vi "UpdateLoadTroque.vi"(8 "error in (no error)":errorcluster, 10 "TorqueValue(%)":dbl, 11 "MFActor in":refnum<class "MFActor.lvclass">) -> (0 "error out":errorcluster, 3 "MFActor out":refnum<class "MFActor.lvclass">)   [LabVIEW 2024, in "MFActor.lvlib" / "MFActor.lvclass"]
uses:
  MFActor.lvclass
  MFActor.lvclass/MFActor.ctl
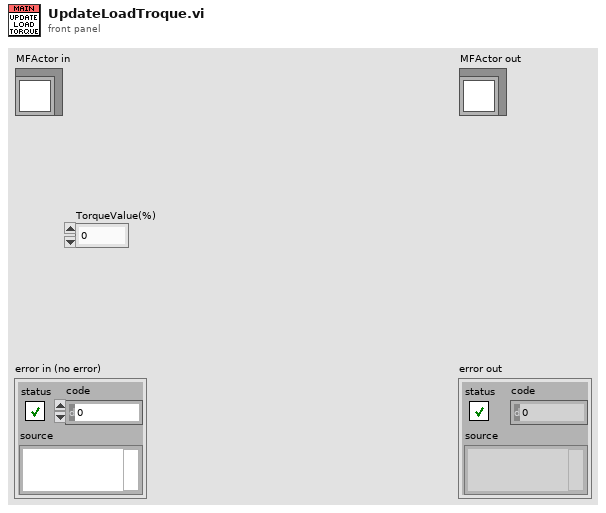
[diagram p1: front panel]
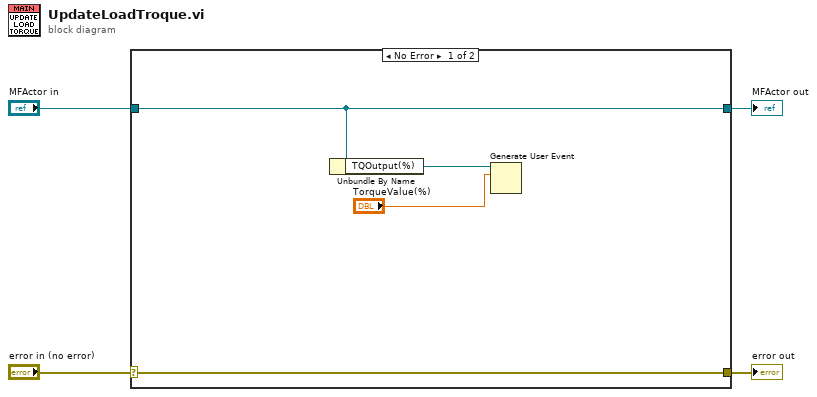
[diagram p0: block diagram]
diagram:
  n1 = case shown="No Error" "error in (no error)" {
    selector: "error in (no error)" -> [w8 w10]
    tunnel: [w8 w10] -> w3
    tunnel: [w7 w9] -> w1
    tunnel: "MFActor in" -> [w7 w9]
    frame No Error {
      n2 = Unbundle By Name(w7) -> ("TQOutput(%)"=w6:refnum<user-event>)
      n3 = Generate User Event(user event=w6, event data cluster="TorqueValue(%)") -> ()  [unwired: 2 in, 2 out]
    }
    frame Error {
    }
  }
  "error out" <- w3
  "MFActor out" <- w1
